vi "ReadHDF5data.vi"() -> ()   [LabVIEW 2014]
uses:
  <vilib>/addons/h5labview2/file/H5Fmode.ctl
  <vilib>/addons/h5labview2/base/lib_path.vi
  <vilib>/addons/h5labview2/base/H5Equery.vi
  <vilib>/addons/h5labview2/dataset/H5Dread.llb/H5Dread.xnode
  <vilib>/addons/h5labview2/file/H5F.lvlib
  <vilib>/addons/h5labview2/group/H5G.lvlib
panel:
  out "# Trigs":i32
  out "# Events in Histo":dbl
  in  "Low Range Threshold":dbl=400.0 format="%#_13g"
  out "Waveform Graph":dbl[](graph)
  in  "Number of Bins":i32=4096
  in  "stop":bool
  out "XY Graph":cluster{sgl[], sgl[]}(graph)
  in  "Channel":u8
  out "raw data":T1(array[cluster])
  in  "File path":path
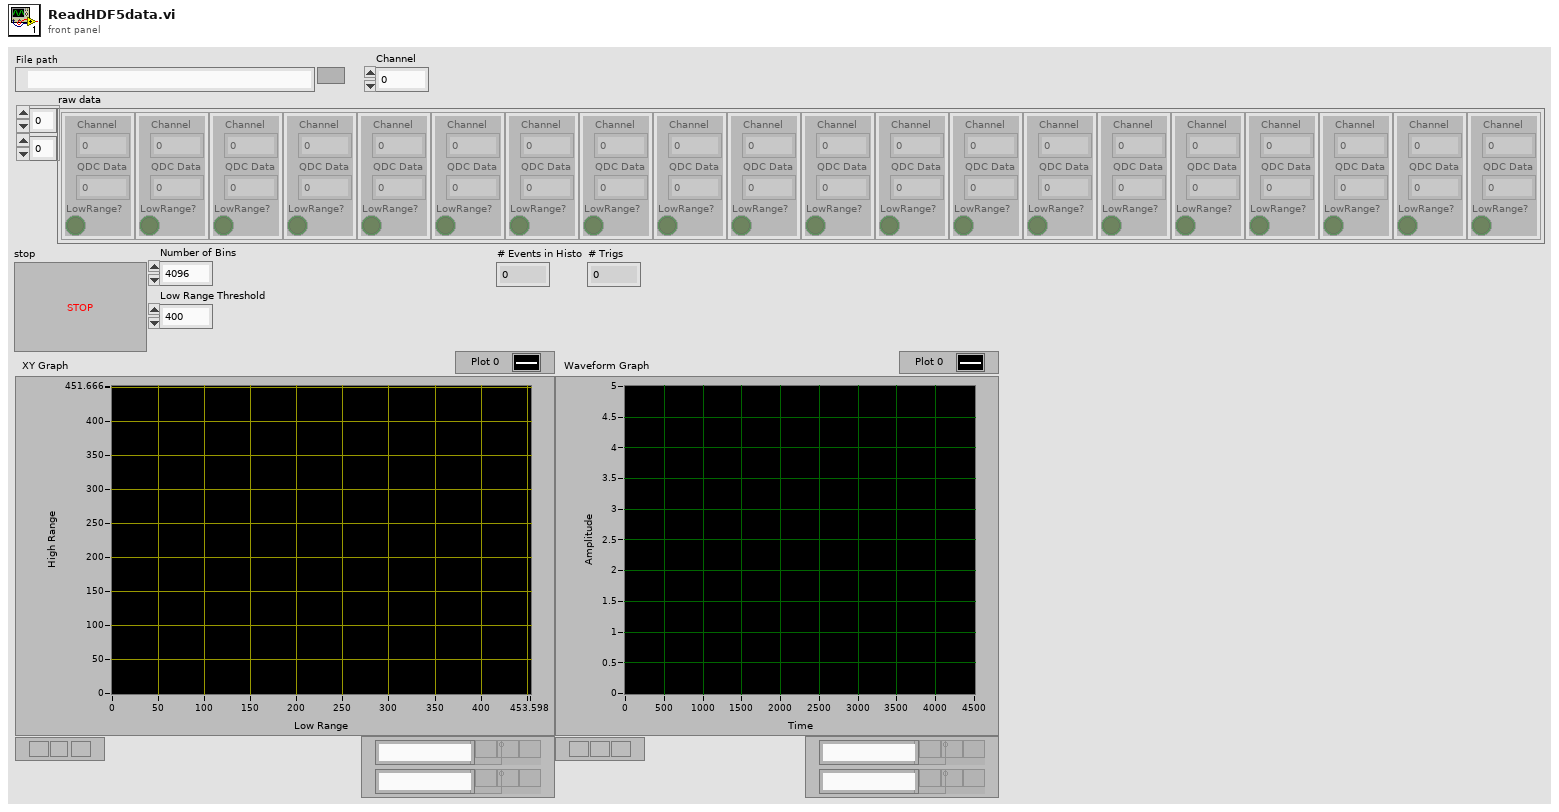
[diagram p1: front panel]
types:
  T1 = cluster{"Channel":u8, "QDC Data":sgl, "LowRange?":bool}[][]
  T2 = typedef "H5F.lvlib/H5Fmode.ctl" = enum16{"read-only", "read-write", "overwrite", "create new", "open or create"}
  T3 = cluster{"Channel":u8, "QDC Data":sgl, "LowRange?":bool}[]
  T4 = typedef "hid_t.ctl" = i32
  T5 = typedef "h5o_type.ctl" = enum8{"Group", "Dataset", "Named type"}
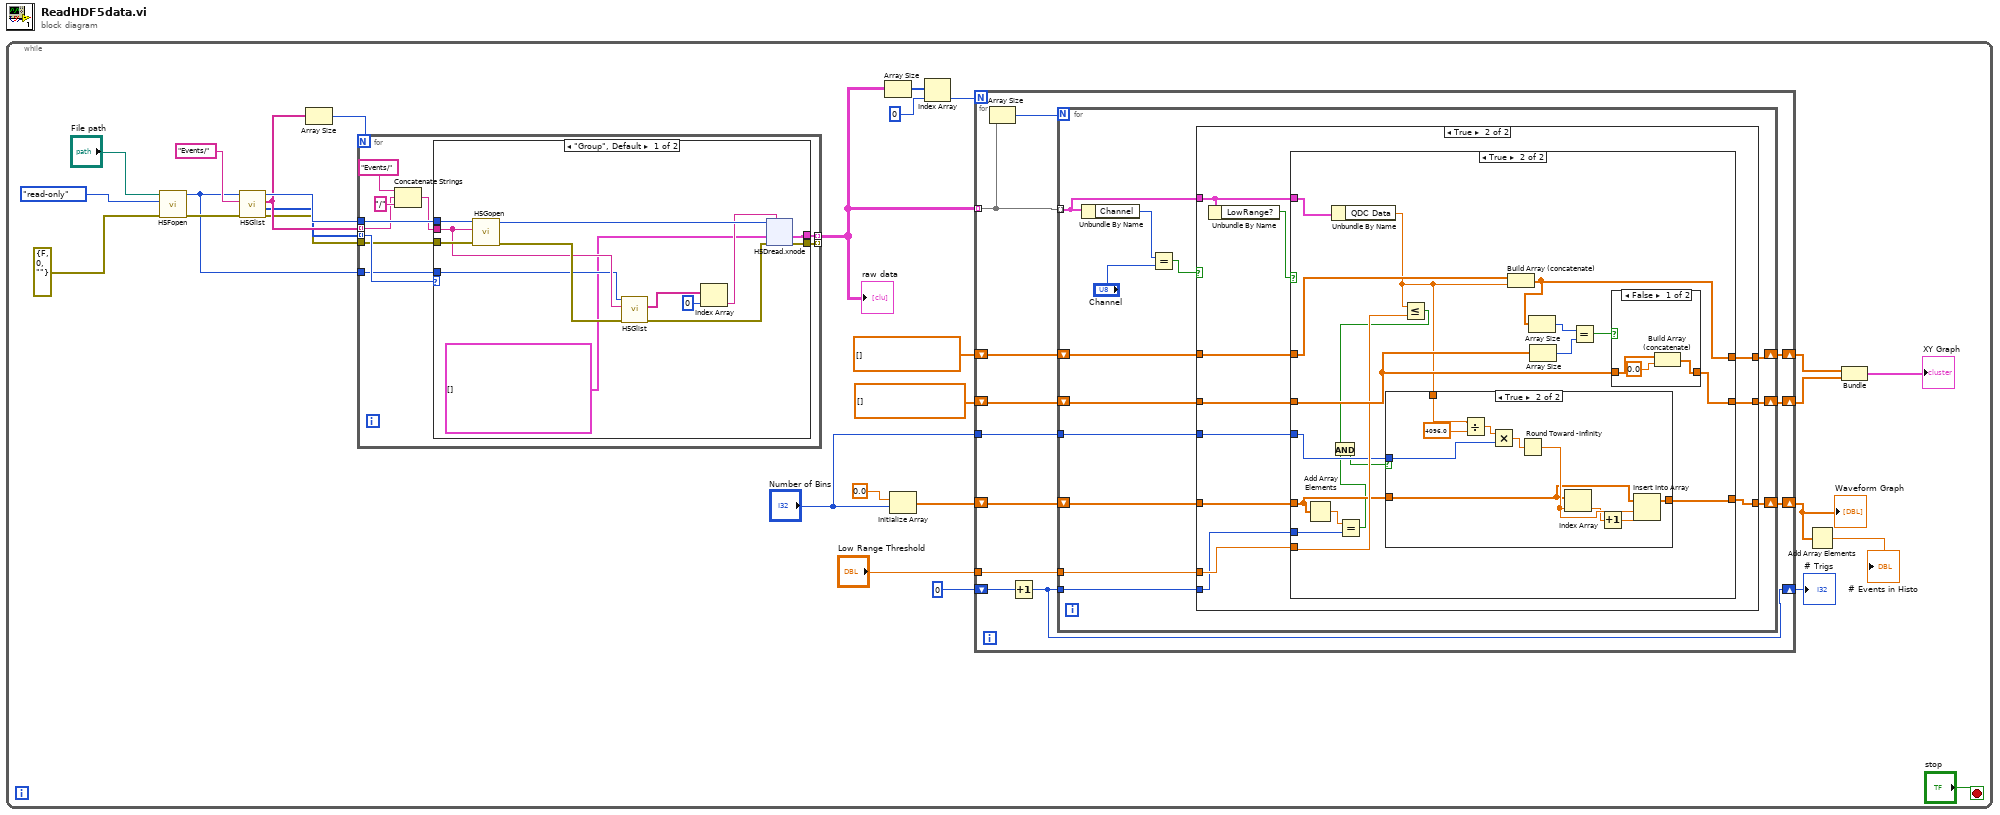
[diagram p0: block diagram]
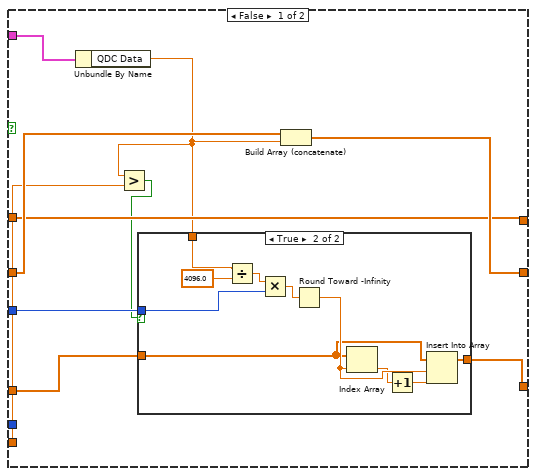
[diagram p3: hidden frame]
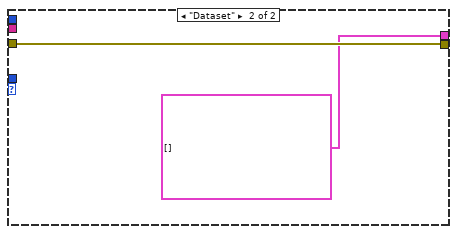
[diagram p7: hidden frame]
diagram:
  n1 = while {
    stop <- "stop" stop-if-true
    n2 = call <vilib>:"H5Fopen.vi"("error in (no error)"=errorcluster {"status"=FALSE, "code"=0, "source"=""}, "mode (read-only)"=H5Fmode."read-only", "path"="File path") -> ("error out"=w26:errorcluster, "ref out"=w19:T4)  [unwired: 7 in]
    n3 = call <vilib>:"H5Glist.vi"("error in (no error)"=w26, "group (.)"="Events/", "ref in"=w19) -> ("error out"=w20:errorcluster, "types"=w21:T5[], "names"=w22:string[], "ref out"=w23:T4)  [unwired: 5 in]
    n4 = Array Size(array=w22) -> (size(s)=w24:i32)
    n5 = for {
      N: w24 -> [_]
      tunnel: w23 -> [w130]
      tunnel: w22 -> [w126] mode=indexing
      tunnel: w21 -> [w132] mode=indexing
      tunnel: w20 -> [w131]
      tunnel: w19 -> [w125]
      tunnel: [w124] -> _ mode=indexing
      tunnel: [w123] -> w15 mode=indexing
      n6 = Concatenate Strings("Events/" ("group (.)"), w126, "/" ("string")) -> (w128:string)
      n7 = case shown="\"Group\", Default" w132 {
        tunnel: w131 -> [w145 w162]
        tunnel: w128 -> [w142 _]
        tunnel: w130 -> [w144 _]
        tunnel: w125 -> [w139 _]
        tunnel: [w134 w162] -> w124
        tunnel: [w133 T3 []] -> w123
        frame "Group", Default {
          n8 = call <vilib>:"H5Gopen.vi"("error in (no error)"=w145, "name"=w142, "ref in"=w144) -> ("error out"=w143:errorcluster, "group out"=w140:T4)  [unwired: 7 in]
          n9 = call <vilib>:"H5Glist.vi"("error in (no error)"=w143, "group (.)"=w142, "ref in"=w139) -> ("error out"=w141:errorcluster, "names"=w138:string[])  [unwired: 5 in, 2 out]
          n10 = Index Array(array=w138, index=0) -> (element=w136:string)
          n11 = xnode "H5Dread.xnode"("dataset name (this)"=w136, "error in (no error)"=w141, "default"=T3 [], "ref in"=w140) -> ("error out"=w134:errorcluster, "data"=w133:T3)  [unwired: 2 in, 2 out]
        }
        frame "Dataset" {
        }
      }
    }
    "raw data" <- w15
    n12 = Array Size(array=w15) -> (size(s)=w18:i32[])
    n13 = Initialize Array(0.0 ("element"), "Number of Bins") -> (w7:dbl[])
    n14 = Index Array(array=w18, index=0) -> (element=w16:i32)
    n15 = for {
      N: w16 -> [_]
      tunnel: w15 -> [w40] mode=indexing
      shift-right: [w37] -> w12
      shift-left: sgl[] [] -> [w39]
      shift-right: [w36] -> w11
      shift-left: sgl[] [] -> [w38]
      shift-right: [w33] -> w3
      shift-left: w7 -> [w35]
      tunnel: "Number of Bins" -> [w34]
      tunnel: "Low Range Threshold" -> [w32]
      shift-right: [w30] -> w1
      shift-left: 0 -> [w31]
      n16 = Array Size(array=w40) -> (size(s)=w41:i32)
      n17 = Increment(x=w31) -> (x+1=w30:i32)
      n18 = for {
        N: w41 -> [_]
        tunnel: w40 -> [w51] mode=indexing
        shift-right: [w47] -> w36
        shift-left: w38 -> [w48]
        shift-right: [w49] -> w37
        shift-left: w39 -> [w50]
        shift-right: [w44] -> w33
        shift-left: w35 -> [w46]
        tunnel: w34 -> [w45]
        tunnel: w32 -> [w43]
        tunnel: w30 -> [w42]
        n19 = Unbundle By Name(w51) -> ("Channel"=w54:u8)
        n20 = Equal?(x=w54, y="Channel") -> (x = y?=w52:bool)
        n21 = case shown="True" w52 {
          tunnel: w51 -> [_ w67]
          tunnel: w50 -> [w57 w66]
          tunnel: [w57 w65] -> w49
          tunnel: w48 -> [w56 w64]
          tunnel: [w56 w63] -> w47
          tunnel: w46 -> [w55 w62]
          tunnel: w45 -> [_ w61]
          tunnel: [w55 w60] -> w44
          tunnel: w43 -> [_ w59]
          tunnel: w42 -> [_ w58]
          frame False {
          }
          frame True {
            n22 = Unbundle By Name(w67) -> ("LowRange?"=w68:bool)
            n23 = case shown="True" w68 {
              tunnel: w67 -> [w78 w107]
              tunnel: w66 -> [w75 w106]
              tunnel: [w75 w105] -> w65
              tunnel: w64 -> [w77 w101]
              tunnel: [w76 w100] -> w63
              tunnel: w62 -> [w73 w93]
              tunnel: w61 -> [w74 w96]
              tunnel: [w72 w99] -> w60
              tunnel: w59 -> [w69 w98]
              tunnel: w58 -> [_ w94]
              frame False {
                n24 = Unbundle By Name(w78) -> ("QDC Data"=w71:sgl)
                n25 = Greater?(x=w71, y=w69) -> (0:w70:bool)
                n26 = case shown="True" w70 {
                  tunnel: w71 -> [_ w89]
                  tunnel: w74 -> [_ w86]
                  tunnel: w73 -> [w79 w83]
                  tunnel: [w79 w80] -> w72
                  frame False {
                  }
                  frame True {
                    n27 = Divide(x=w89, y=sgl 4096.0) -> (x/y=w87:sgl)
                    n28 = Multiply(x=w87, y=w86) -> (x*y=w85:sgl)
                    n29 = Round Toward -Infinity(1:w85) -> (0:w84:sgl)
                    n30 = Index Array(array=w83, index=w84) -> (element=w81:dbl)
                    n31 = Increment(x=w81) -> (x+1=w82:dbl)
                    n32 = Insert Into Array(array=w83, index=w84, new element=w82) -> (w80:dbl[])
                  }
                }
                n33 = Build Array (concatenate)(w77, w71) -> (w76:sgl[])
              }
              frame True {
                n34 = Add Array Elements(numeric array=w93) -> (sum=w92:dbl)
                n35 = Unbundle By Name(w107) -> ("QDC Data"=w95:sgl)
                n36 = Equal?(x=w92, y=w94) -> (x = y?=w90:bool)
                n37 = Less Or Equal?(x=w95, y=w98) -> (x <= y?=w97:bool)
                n38 = And(x=w97, y=w90) -> (x .and. y?=w91:bool)
                n39 = case shown="True" w91 {
                  tunnel: w95 -> [_ w118]
                  tunnel: w96 -> [_ w115]
                  tunnel: w93 -> [w108 w112]
                  tunnel: [w108 w109] -> w99
                  frame False {
                  }
                  frame True {
                    n40 = Divide(x=w118, y=sgl 4096.0) -> (x/y=w116:sgl)
                    n41 = Multiply(x=w116, y=w115) -> (x*y=w114:sgl)
                    n42 = Round Toward -Infinity(1:w114) -> (0:w113:sgl)
                    n43 = Index Array(array=w112, index=w113) -> (element=w110:dbl)
                    n44 = Increment(x=w110) -> (x+1=w111:dbl)
                    n45 = Insert Into Array(array=w112, index=w113, new element=w111) -> (w109:dbl[])
                  }
                }
                n46 = Build Array (concatenate)(w106, w95) -> (w105:sgl[])
                n47 = Array Size(array=w105) -> (size(s)=w103:i32)
                n48 = Array Size(array=w101) -> (size(s)=w102:i32)
                n49 = Equal?(x=w103, y=w102) -> (x = y?=w104:bool)
                n50 = case shown="False" w104 {
                  tunnel: w101 -> [w121 w122]
                  tunnel: [w119 w122] -> w100
                  frame False {
                    n51 = Build Array (concatenate)(w121, sgl 0.0 ("High Range Data")) -> (w119:sgl[])
                  }
                  frame True {
                  }
                }
              }
            }
          }
        }
      }
    }
    "Waveform Graph" <- w3
    "# Trigs" <- w1
    n52 = Add Array Elements(numeric array=w3) -> (sum=→"# Events in Histo":dbl)
    n53 = Bundle(w12, w11) -> (→"XY Graph":cluster{sgl[], sgl[]})  [unwired: 1 in]
  }
